vi "APTget.vi"(8 "error in (no error)":errorcluster, 11 "reference":refnum<k7>) -> (0 "error out":errorcluster, 2 "pfPosition":sgl, 3 "reference out":refnum<k7>)   [LabVIEW 2013]
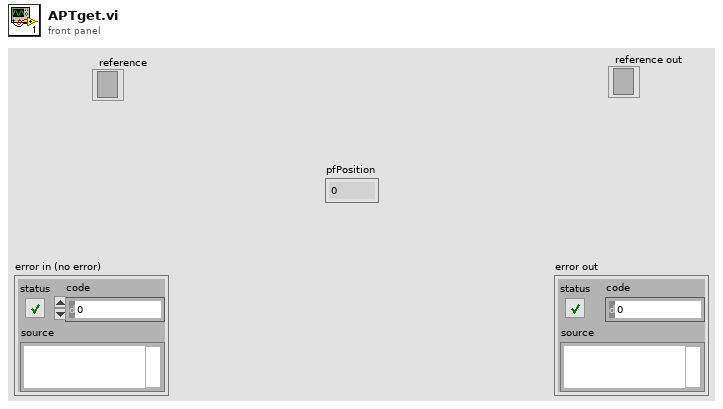
[diagram p1: front panel]
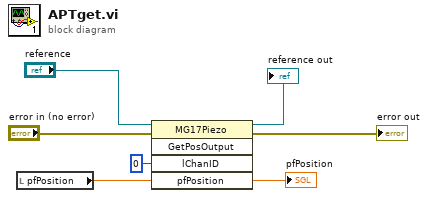
[diagram p0: block diagram]
diagram:
  n1 = local read "pfPosition"() -> (w1:sgl)
  n2 = invoke class="MG17Piezo" method="GetPosOutput"(reference="reference", error in="error in (no error)", "lChanID"=0, "pfPosition"=w1) -> (reference out=→"reference out":refnum<k7>, error out=→"error out":errorcluster, "pfPosition"=→"pfPosition":sgl)  [unwired: 1 in, 2 out]
